vi "Histogram Based Min and Max.vi"(10 "Data to Histogram":sgl[](array[numeric]), 11 "Histogram Graph":T1) -> (3 "Histogram Properties":cluster{"Min":sgl, "Max":sgl})   [LabVIEW 2014]
uses:
  <vilib>/Analysis/6fits.llb/Curve Fitting Criteria.ctl
  <vilib>/Analysis/NI_AALBase.lvlib
  <vilib>/Analysis/NI_AALPro.lvlib
panel:
  out "Waveform Graph":dbl[][](graph)
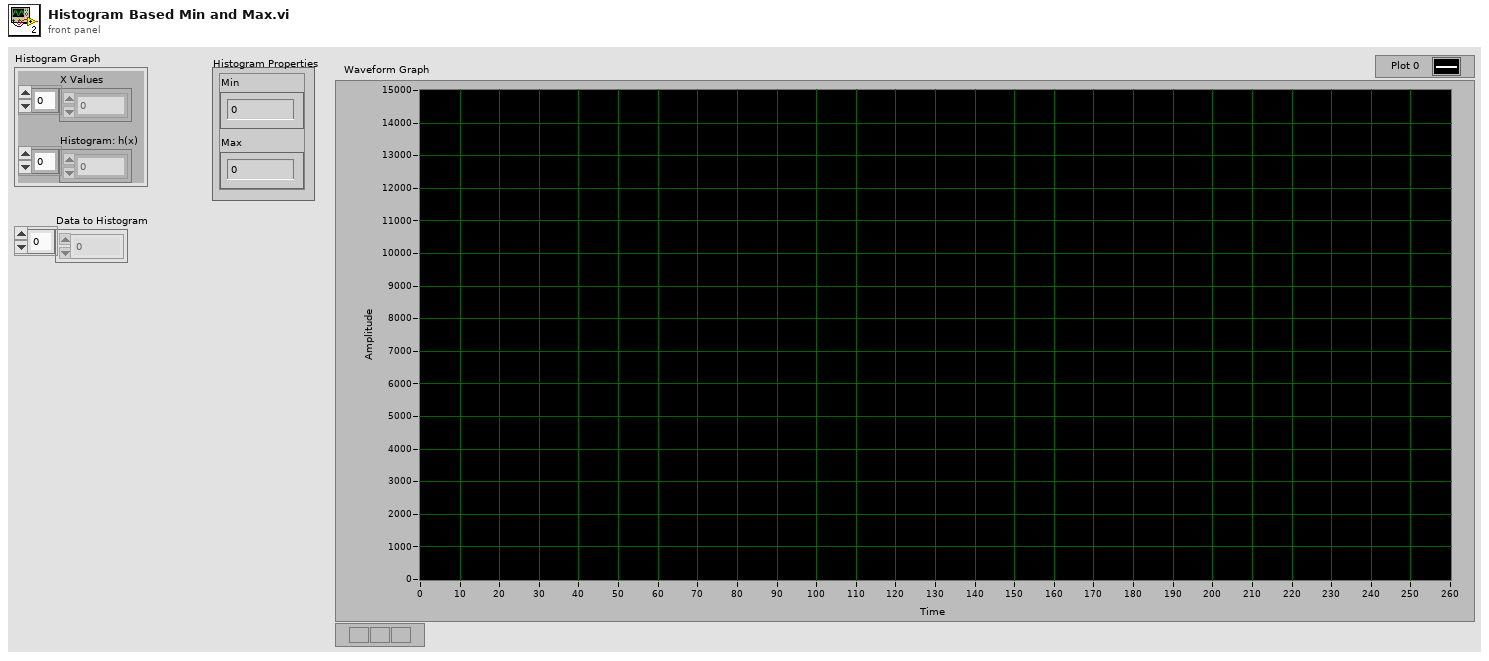
[diagram p1: front panel]
types:
  T1 = cluster{"X Values":dbl[], "Histogram: h(x)":i32[]}
  T2 = typedef "NI_AALPro.lvlib/Curve Fitting Criteria.ctl" = u16
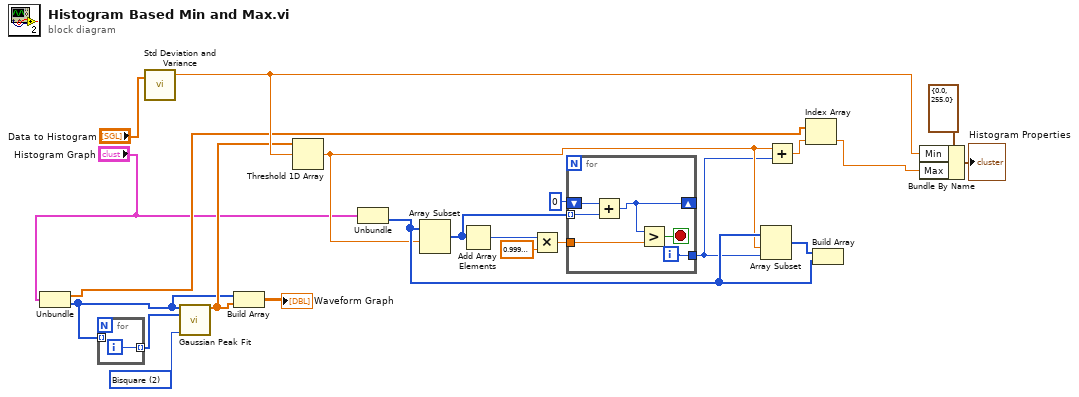
[diagram p0: block diagram]
diagram:
  w7 = T2 2 items=["Least Square", "Least Absolute Residual", "Bisquare"] ("method")
  n1 = Unbundle("Histogram Graph") -> ("X Values"=w4:dbl[], "Histogram: h(x)"=w5:i32[])
  n2 = for {
    tunnel: [w23] -> w8 mode=indexing
    tunnel: w5 -> [_] mode=indexing
    i -> [w23]
  }
  n3 = call <vilib>:"Std Deviation and Variance.vi"("X"="Data to Histogram") -> ("mean"=w16:dbl)  [unwired: 1 in, 2 out]
  n4 = call <vilib>:"Gaussian Peak Fit.vi"("Y"=w5, "X"=w8, "method"=w7) -> ("Best Gaussian Fit"=w6:dbl[])  [unwired: 6 in, 6 out]
  n5 = Build Array(w5, w6) -> (→"Waveform Graph":dbl[][])
  n6 = Threshold 1D Array(2:w16, 3:w6) -> (0:w10:dbl)  [unwired: 1 in]
  n7 = Unbundle("Histogram Graph") -> ("Histogram: h(x)"=w13:i32[])  [unwired: 1 out]
  n8 = Array Subset(array=w13, index=w10) -> (w15:i32[])  [unwired: 1 in]
  n9 = Add Array Elements(numeric array=w15) -> (sum=w18:i32)
  n10 = Multiply(x=w18, y=sgl 0.999) -> (x*y=w17:sgl)
  n11 = for {
    tunnel: w15 -> [w29] mode=indexing
    shift-right: [w27] -> _
    shift-left: 0 -> [w28]
    tunnel: [w25] -> w9
    tunnel: w17 -> [w24]
    i -> [w25]
    stop <- w26 stop-if-true
    n12 = Add(x=w28, y=w29) -> (x+y=w27:i32)
    n13 = Greater?(x=w27, y=w24) -> (0:w26:bool)
  }
  n14 = Array Subset(array=w13, index=w10, length=w9) -> (w14:i32[])
  n15 = Add(x=w10, y=w9) -> (x+y=w11:dbl)
  n16 = Index Array(array=w4, index=w11) -> (element=w12:dbl)
  n17 = Build Array(w14, w13) -> ()  [unwired: 1 out]
  n18 = Bundle By Name(cluster=cluster{"Min":sgl, "Max":sgl} {"Min"=0.0, "Max"=255.0} ("Histogram Properties"), "Min"=w16, "Max"=w12) -> (→"Histogram Properties":cluster{"Min":sgl, "Max":sgl})
